vi "RT_Thrust_Force_in_DLR_Body_Reference_System(SubVI).vi"(6 "Act_b(i)":dbl[](array[numeric]), 8 "Nzl_S":dbl, 9 "i":i32, 10 "Patm (Pa)":dbl, 11 "Data":dbl[][](array[numeric])) -> (3 "FE_b":dbl[](array[numeric]))   [LabVIEW 2017]
panel:
  out "Fez":dbl
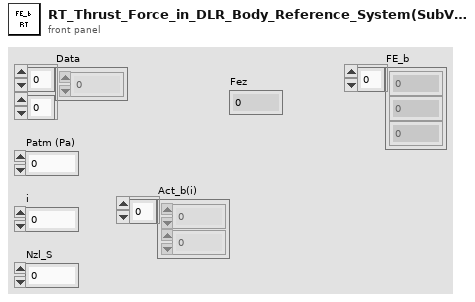
[diagram p1: front panel]
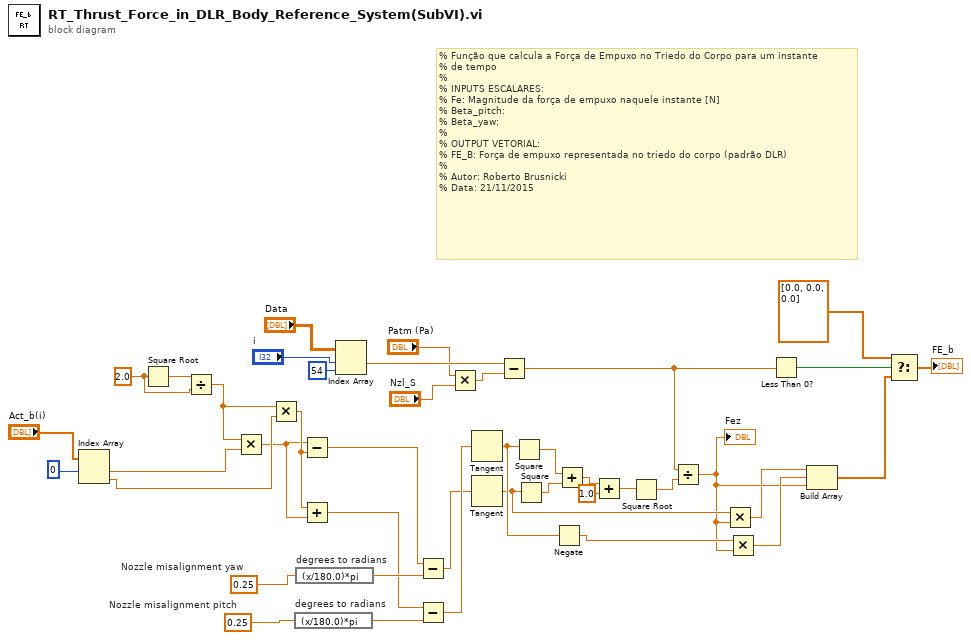
[diagram p0: block diagram]
diagram:
  w10 = 2.0 ("x")
  w13 = 0.25  # Nozzle misalignment pitch
  w12 = 0.25  # Nozzle misalignment yaw
  # "% Função que calcula a Força de Empuxo no Triedo do Corpo para um instante\n% de tempo\n%\n% INPUTS ESCALARES:\n% Fe: Magnitude da força de empuxo naquele instante [N]\n% Beta_pitch: \n% Beta_yaw:\n%\n% OUTPUT VETORIAL:\n% FE_B: Força de empuxo representada no triedo do corpo (padrão DLR)\n%\n% Autor: Roberto Brusnicki\n% Data: 21/11/2015"
  n1 = Index Array(array="Act_b(i)", index #1=0 ("disabled index (col)")) -> (element #1=w9:dbl, element #2=w7:dbl)  [unwired: 1 in]
  n2 = Square Root(x=w10) -> (sqrt(x)=w11:dbl)
  n3 = Divide(x=w11, y=w10) -> (x/y=w8:dbl)
  n4 = Multiply(x=w8, y=w9) -> (x*y=w4:dbl)
  n5 = Multiply(x=w8, y=w7) -> (x*y=w5:dbl)
  n6 = expression code="(x/180.0)*pi" "degrees to radians"(w13) -> (w14:dbl)
  n7 = expression code="(x/180.0)*pi" "degrees to radians"(w12) -> (w15:dbl)
  n8 = Subtract(x=w4, y=w5) -> (x-y=w6:dbl)
  n9 = Add(x=w5, y=w4) -> (x+y=w3:dbl)
  n10 = Index Array(array="Data", index (row)="i", index (col)=54 ("disabled index (col)")) -> (element=w31:dbl)
  n11 = Subtract(x=w6, y=w15) -> (x-y=w1:dbl)
  n12 = Subtract(x=w3, y=w14) -> (x-y=w2:dbl)
  n13 = Multiply(x="Patm (Pa)", y="Nzl_S") -> (x*y=w24:dbl)
  n14 = Tangent(1:w2) -> (0:w36:dbl)
  n15 = Tangent(1:w1) -> (0:w35:dbl)
  n16 = Subtract(x=w31, y=w24) -> (x-y=w18:dbl)
  n17 = Square(x=w36) -> (x^2=w27:dbl)
  n18 = Square(x=w35) -> (x^2=w26:dbl)
  n19 = Negate(x=w36) -> (-x=w37:dbl)
  n20 = Add(x=w27, y=w26) -> (x+y=w28:dbl)
  n21 = Add(x=w28, y=1.0) -> (x+y=w30:dbl)
  n22 = Square Root(x=w30) -> (sqrt(x)=w32:dbl)
  n23 = Divide(x=w18, y=w32) -> (x/y=w34:dbl)
  "Fez" <- w34
  n24 = Multiply(x=w35, y=w34) -> (x*y=w33:dbl)
  n25 = Multiply(x=w37, y=w34) -> (x*y=w38:dbl)
  n26 = Less Than 0?(x=w18) -> (x < 0?=w25:bool)
  n27 = Build Array(w33, w38, w34) -> (w40:dbl[])
  n28 = Select(t=dbl[] [0.0, 0.0, 0.0], s=w25, f=w40) -> (s? t:f=→"FE_b":dbl[])
